vi "sv_Check Maximum Harmonic and Mapping.vi"(1 "harmonics to visualize in":i32[](array[numeric]), 11 "error in (no error)":errorcluster, 12 "maximum harmonic in":i32) -> (3 "dup harmonics to visualize":i32[](array[numeric]), 14 "dup maximum harmonic":i32, 15 "error out":errorcluster)   [LabVIEW 2017, in "SoundVib_Distortion.lvlib"]
uses:
  <vilib>/addons/Sound and Vibration/svt_Distortion/SoundVib_Distortion.lvlib
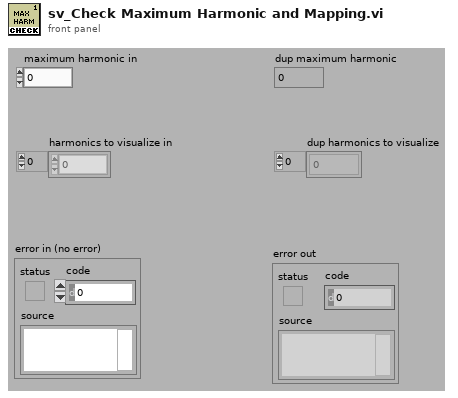
[diagram p1: front panel]
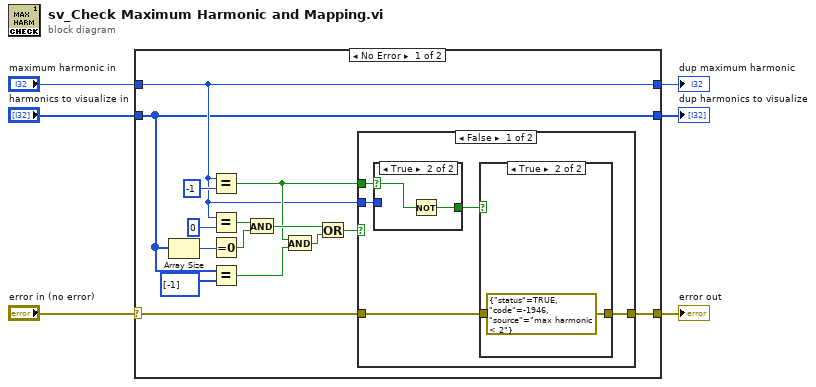
[diagram p0: block diagram]
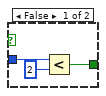
[diagram p2: hidden frame]
diagram:
  n1 = case shown="No Error" "error in (no error)" {
    selector: "error in (no error)" -> [w21 w37]
    tunnel: [w20 w37] -> w5
    tunnel: "maximum harmonic in" -> [w8 w35]
    tunnel: "harmonics to visualize in" -> [w7 w36]
    tunnel: [w7 w36] -> w2
    tunnel: [w8 w35] -> w4
    frame No Error {
      n2 = Array Size(array=w7) -> (size(s)=w18:i32)
      n3 = Equal?(x=w8, y=-1) -> (x = y?=w11:bool)
      n4 = Equal?(x=w8, y=0 ("x")) -> (x = y?=w17:bool)
      n5 = Equal To 0?(x=w18) -> (x = 0?=w19:bool)
      n6 = Equal?(x=w7, y=i32[] [-1] ("harmonics to visualize in")) -> (x = y?=w9:bool)
      n7 = And(x=w17, y=w19) -> (x .and. y?=w14:bool)
      n8 = And(x=w11, y=w9) -> (x .and. y?=w13:bool)
      n9 = Or(x=w14, y=w13) -> (x .or. y?=w12:bool)
      n10 = case shown="False" w12 {
        tunnel: w21 -> [w26 w34]
        tunnel: [w25 w34] -> w20
        tunnel: w8 -> [w24 _]
        tunnel: w11 -> [w22 _]
        frame False {
          n11 = case shown="True" w22 {
            selector: w22 -> [_ w31]
            tunnel: [w29 w30] -> w23
            tunnel: w24 -> [w27 _]
            frame False {
              n12 = Less?(x=w27, y=2 ("lower limit")) -> (x < y?=w29:bool)
            }
            frame True {
              n13 = Not(x=w31) -> (.not. x?=w30:bool)
            }
          }
          n14 = case shown="True" w23 {
            tunnel: w26 -> [w32 _]
            tunnel: [w32 errorcluster {"status"=TRUE, "code"=-1946, "source"="max harmonic < 2"} ("error IO")] -> w25
            frame False {
            }
            frame True {
            }
          }
        }
        frame True {
        }
      }
    }
    frame Error {
    }
  }
  "error out" <- w5
  "dup maximum harmonic" <- w4
  "dup harmonics to visualize" <- w2
